vi "Conditional Increment - Double.vi"(2 "Condition":bool, 3 "Input":dbl) -> (0 "Output":dbl)   [LabVIEW 2013, in "femtoRoboLib.lvlib"]
uses:
  femtoRoboLib.lvlib
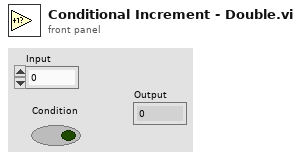
[diagram p1: front panel]
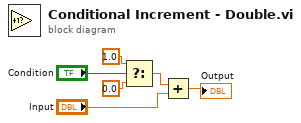
[diagram p0: block diagram]
diagram:
  n1 = Select(t=1.0, s="Condition", f=0.0 ("t")) -> (s? t:f=w4:dbl)
  n2 = Add(x=w4, y="Input") -> (x+y=→"Output":dbl)
